vi "Launch Class.vi"() -> ()   [LabVIEW 2016]
uses:
  <vilib>/Utility/miscctls.llb/LVRectTypeDef.ctl
  <vilib>/Utility/miscctls.llb/LVPositionTypeDef.ctl
  <vilib>/Utility/miscctls.llb/LVBoundsTypeDef.ctl
  <vilib>/Utility/miscctls.llb/LVPointTypeDef.ctl
panel:
  out "Pane: Origin":T1
  out "Panel: TotalRectangle":T2
  out "Panel: Master Rectangle":T2
  out "Panel: Bounds":T3
  out "Pane: Position":T4
  out "Pane: Bounds":T3
  out "VI: FrontPanel.WindowBounds":T2
  out "Control: Position":T4
  out "Control: Master Bounds Rect":T2
  out "Control: Total Bounds Rect":T2
  out "Pane: Content Area Rect":T2
  out "VI: FrontPanel.PanelBounds":T2
  in  "Stop":bool
  # "Window bounds are the rectangle of monitor-based coordinates. \n.... In Windows 10 these seem to be a little off on the sides.\n\nPanel bounds remove the title bar, scroll bars, etc.\n\nMove the VI Front Panel window around to see these change."
  # "Panel Bounds: Changes as objects are moved. Bounding \nrectangle?\n\nPanel Master Rectangle: Always has Left = 0, Top = 46. Right and\nBottom change as window is resized.  \n\nTotal Rectangle:  cxczx"
  # "Content Area Rect: Left and Top are same as Origin: Horz and\nOrigin: Vert. \n\nPane Bounds: Changes as window is resized. Seems connected to \nPanel Master Rectangle\n\nPosition: Top Left Coordinates of rectangle bounding all objects relative to gray dot. \n\nOrigin: Coordinates of the upper left corner relative to the gray dot.\nIf the gray dot is visible, these will always be negative."
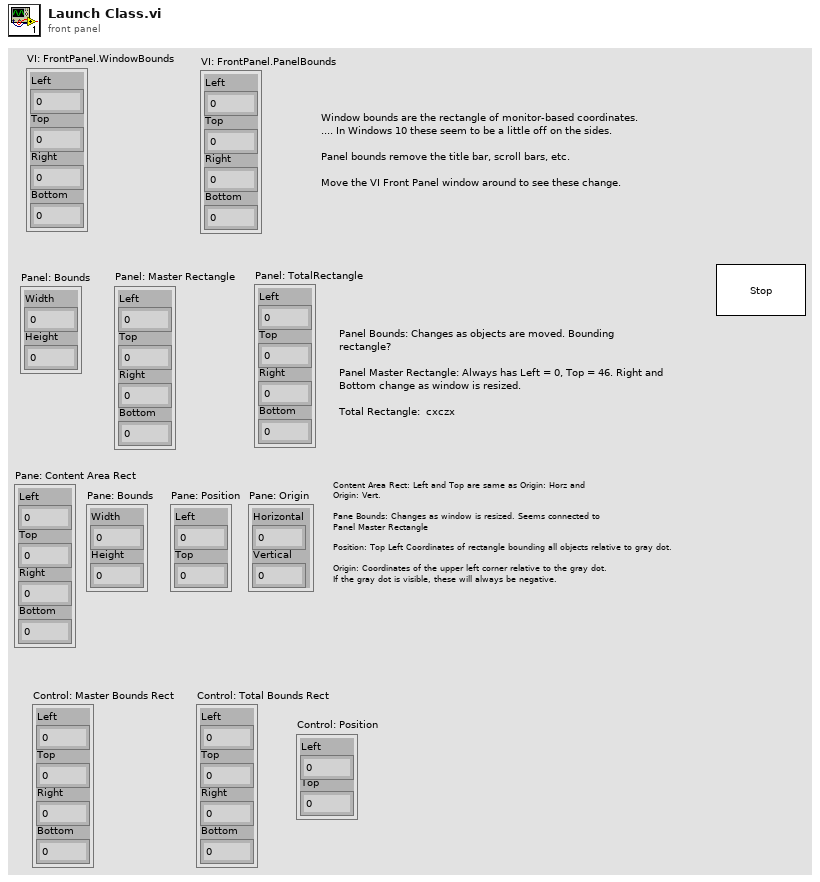
[diagram p1: front panel]
types:
  T1 = typedef "LVPointTypeDef.ctl" = cluster{"Horizontal":i16, "Vertical":i16}
  T2 = typedef "LVRectTypeDef.ctl" = cluster{"Left":i16, "Top":i16, "Right":i16, "Bottom":i16}
  T3 = typedef "LVBoundsTypeDef.ctl" = cluster{"Width":u32, "Height":u32}
  T4 = typedef "LVPositionTypeDef.ctl" = cluster{"Left":i32, "Top":i32}
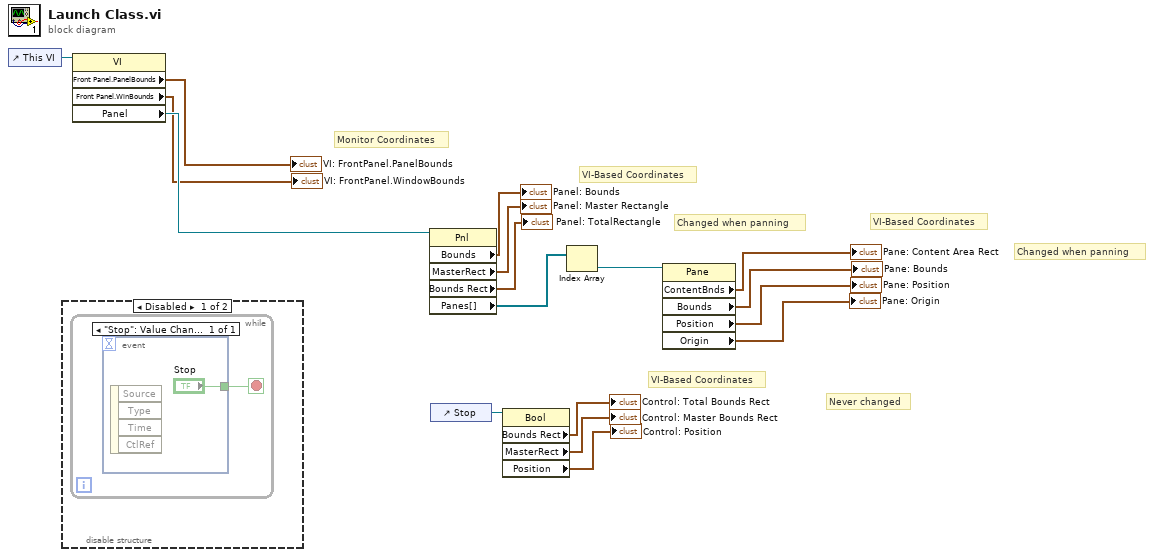
[diagram p0: block diagram]
diagram:
  # "Never changed"
  # "Changed when panning"
  # "Changed when panning"
  # "VI-Based Coordinates"
  # "VI-Based Coordinates"
  # "VI-Based Coordinates"
  # "Monitor Coordinates"
  n1 = control-ref of="This VI"() -> (w17:refnum<vi>)
  n2 = disable-structure shown="Disabled" {
    frame Disabled {
      n3 = while {
        stop <- w18 stop-if-true
        n4 = event shown="[0] \"Stop\": Value Change" {
          selector: _ -> [_]
          dyn-events: _ -> [_]
          timeout: _ -> [_]
          tunnel: ["Stop"] -> w18
          event "Stop": Value Change {
            n5 = event-data() -> ()  [unwired: 1 in, 4 out]
          }
        }
      }
    }
    frame Enabled {
    }
  }
  n6 = property class="VI"(reference=w17) -> ("Front Panel.PanelBounds"=→"VI: FrontPanel.PanelBounds":T2, "Front Panel.WinBounds"=→"VI: FrontPanel.WindowBounds":T2, "Panel"=w15:refnum<vi>)  [unwired: 1 in, 2 out]
  n7 = property class="Pnl"(reference=w15) -> ("Bounds"=→"Panel: Bounds":T3, "MasterRect"=→"Panel: Master Rectangle":T2, "Bounds Rect"=→"Panel: TotalRectangle":T2, "Panes[]"=w5:refnum<vi>[])  [unwired: 1 in, 2 out]
  n8 = control-ref of="Stop"() -> (w12:refnum<vi>)
  n9 = property class="Bool"(reference=w12) -> ("Bounds Rect"=→"Control: Total Bounds Rect":T2, "MasterRect"=→"Control: Master Bounds Rect":T2, "Position"=→"Control: Position":T4)  [unwired: 1 in, 2 out]
  n10 = Index Array(array=w5) -> (element=w14:refnum<vi>)  [unwired: 1 in]
  n11 = property class="Pane"(reference=w14) -> ("ContentBnds"=→"Pane: Content Area Rect":T2, "Bounds"=→"Pane: Bounds":T3, "Position"=→"Pane: Position":T4, "Origin"=→"Pane: Origin":T1)  [unwired: 1 in, 2 out]
